vi "Read Server Hello.vi"(4 "Port":u16, 6 "Address":string, 8 "error in (no error)":errorcluster, 9 "EventLogger":refnum<class "EventLoggingService.lvclass">, 11 "TCP in":refnum<k5>) -> (0 "error out":errorcluster, 2 "status":T1, 3 "TCP":refnum<k5>)   [LabVIEW 2020, in "Vecto.lvlib" / "TCPMessaging.lvclass"]
uses:
  TCPMessaging.lvclass
  EventLoggingService/EventLoggingService.lvclass
  proto/ConnectStatus/Enumeration.ctl
  EventLoggingService/EventLoggingService.lvclass/EventLoggingService.ctl
  EventLogHandler/EventLogHandler.lvclass
  TCPMessaging.lvclass/TCPMessaging.ctl
  proto/TcpServerHello/TcpServerHello.lvlib
  proto/ConnectStatus/ConnectStatus.lvlib
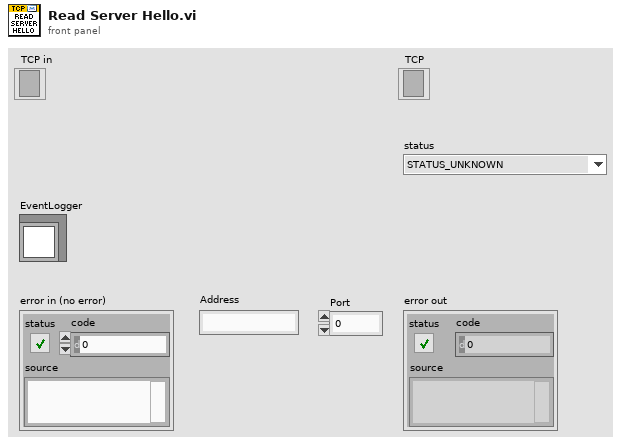
[diagram p1: front panel]
types:
  T1 = typedef "ConnectStatus.lvlib/Enumeration.ctl" = enum16{"STATUS_UNKNOWN", "STATUS_SUCCESS", "STATUS_ERROR", "STATUS_BAD_CONFIG", "STATUS_BAD_SYSTEM", "STATUS_BAD_CLUSTER", "STATUS_NOT_ALLOWED"}
  T2 = typedef "TcpServerHello.lvlib/Data.ctl" = cluster{"status":T1}
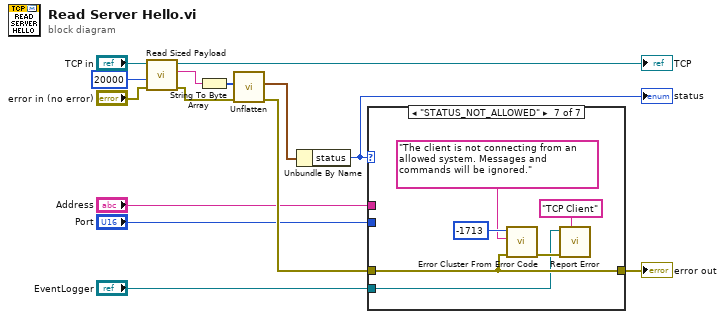
[diagram p0: block diagram]
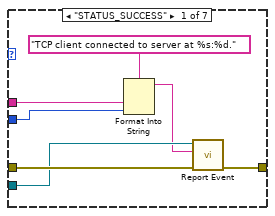
[diagram p2: hidden frame]
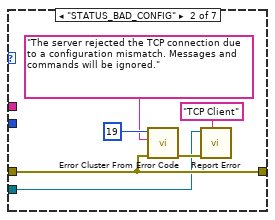
[diagram p3: hidden frame]
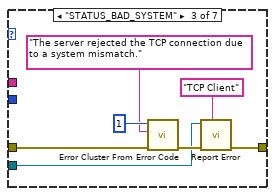
[diagram p4: hidden frame]
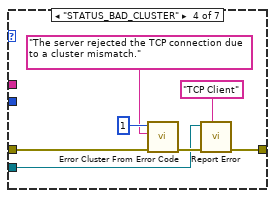
[diagram p5: hidden frame]
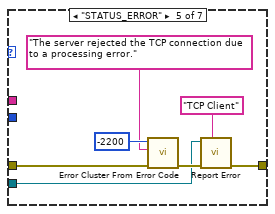
[diagram p6: hidden frame]
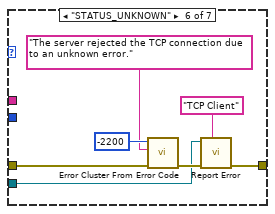
[diagram p7: hidden frame]
diagram:
  n1 = call "Read Sized Payload.vi"("error in (no error)"="error in (no error)", "timeout ms (100)"=20000, "TCP in"="TCP in") -> ("error out"=w8:errorcluster, "Payload"=w10:string, "TCP"=→"TCP":refnum<k5>)  [unwired: 6 in]
  n2 = String To Byte Array(string=w10) -> (unsigned byte array=w9:u8[])
  n3 = call "Unflatten.vi"("error in"=w8, "Buffer"=w9) -> ("error out"=w5:errorcluster, "Data"=w7:T2)  [unwired: 8 in]
  n4 = Unbundle By Name(w7) -> ("status"=w6:T1)
  "status" <- w6
  n5 = case shown="\"STATUS_NOT_ALLOWED\"" w6 {
    tunnel: w5 -> [w21 w27 w34 w41 w48 w55 w61]
    tunnel: [w19 w27 w28 w35 w42 w49 w61] -> w4
    tunnel: "EventLogger" -> [w20 w22 w29 w36 w43 w50 w56]
    tunnel: "Address" -> [w17 _ _ _ _ _ _]
    tunnel: "Port" -> [w16 _ _ _ _ _ _]
    frame "STATUS_SUCCESS" {
      n6 = Format Into String(format string="TCP client connected to server at %s:%d." ("Message"), w17, w16) -> (resulting string=w15:string)  [unwired: 2 in, 1 out]
      n7 = call "Report Event.vi"("error in (no error)"=w21, "Message"=w15, "EventLoggingService in"=w20) -> ("error out"=w19:errorcluster)  [unwired: 7 in, 1 out]
    }
    frame "STATUS_BAD_CONFIG" {
      n8 = call <vilib>:"Error Cluster From Error Code.vi"("error in (no error)"=w27, "error message (\"\")"="The server rejected the TCP connection due to a configuration mismatch. Messages and commands will be ignored.", "error code (0)"=19) -> ("error out"=w24:errorcluster)  [unwired: 6 in]
      n9 = call "Report Error.vi"("Context (None)"="TCP Client", "error in (no error)"=w24, "EventLoggingService in"=w22) -> ()  [unwired: 7 in, 2 out]
    }
    frame "STATUS_BAD_SYSTEM" {
      n10 = call <vilib>:"Error Cluster From Error Code.vi"("error in (no error)"=w34, "error message (\"\")"="The server rejected the TCP connection due to a system mismatch.", "error code (0)"=1) -> ("error out"=w31:errorcluster)  [unwired: 6 in]
      n11 = call "Report Error.vi"("Context (None)"="TCP Client", "error in (no error)"=w31, "EventLoggingService in"=w29) -> ("error out"=w28:errorcluster)  [unwired: 7 in, 1 out]
    }
    frame "STATUS_BAD_CLUSTER" {
      n12 = call <vilib>:"Error Cluster From Error Code.vi"("error in (no error)"=w41, "error message (\"\")"="The server rejected the TCP connection due to a cluster mismatch.", "error code (0)"=1) -> ("error out"=w38:errorcluster)  [unwired: 6 in]
      n13 = call "Report Error.vi"("Context (None)"="TCP Client", "error in (no error)"=w38, "EventLoggingService in"=w36) -> ("error out"=w35:errorcluster)  [unwired: 7 in, 1 out]
    }
    frame "STATUS_ERROR" {
      n14 = call <vilib>:"Error Cluster From Error Code.vi"("error in (no error)"=w48, "error message (\"\")"="The server rejected the TCP connection due to a processing error.", "error code (0)"=-2200) -> ("error out"=w45:errorcluster)  [unwired: 6 in]
      n15 = call "Report Error.vi"("Context (None)"="TCP Client", "error in (no error)"=w45, "EventLoggingService in"=w43) -> ("error out"=w42:errorcluster)  [unwired: 7 in, 1 out]
    }
    frame "STATUS_UNKNOWN" {
      n16 = call <vilib>:"Error Cluster From Error Code.vi"("error in (no error)"=w55, "error message (\"\")"="The server rejected the TCP connection due to an unknown error.", "error code (0)"=-2200) -> ("error out"=w52:errorcluster)  [unwired: 6 in]
      n17 = call "Report Error.vi"("Context (None)"="TCP Client", "error in (no error)"=w52, "EventLoggingService in"=w50) -> ("error out"=w49:errorcluster)  [unwired: 7 in, 1 out]
    }
    frame "STATUS_NOT_ALLOWED" {
      n18 = call <vilib>:"Error Cluster From Error Code.vi"("error in (no error)"=w61, "error message (\"\")"="The client is not connecting from an allowed system. Messages and commands will be ignored.", "error code (0)"=-1713) -> ("error out"=w58:errorcluster)  [unwired: 6 in]
      n19 = call "Report Error.vi"("Context (None)"="TCP Client", "error in (no error)"=w58, "EventLoggingService in"=w56) -> ()  [unwired: 7 in, 2 out]
    }
  }
  "error out" <- w4
